vi "GetAllBooleanControls.vi"(8 "error in (no error)":errorcluster, 11 "VI in":refnum<vi>) -> (0 "error out":errorcluster, 3 "Boolean Controls":refnum<vi>[](array[refnum]))   [LabVIEW 2018, in "CarWashTestCases.lvclass"]
uses:
  CarWashTestCases.lvclass
  <vilib>/Utility/traverseref.llb/TRef TravTarget.ctl
  <vilib>/Utility/traverseref.llb/VI Scripting - Traverse.lvlib
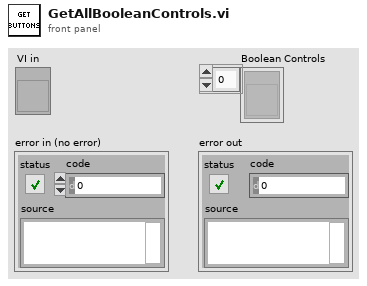
[diagram p1: front panel]
types:
  T1 = typedef "TRef TravTarget.ctl" = enum16{"FP", "BD", "Other"}
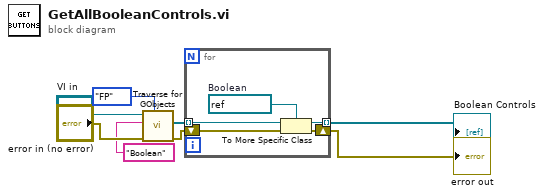
[diagram p0: block diagram]
diagram:
  n1 = call <vilib>:"Traverse for GObjects.vi"("Traverse Target"=TRef_TravTarget."FP", "error in (no error)"="error in (no error)", "Class Name"="Boolean", "VI Refnum"="VI in") -> ("error out"=w7:errorcluster, "References"=w4:refnum<vi>[])  [unwired: 4 in, 2 out]
  n2 = for {
    tunnel: w4 -> [w11] mode=indexing
    tunnel: [w12] -> w5 mode=indexing
    shift-right: [w9] -> w8
    shift-left: w7 -> [w10]
    w13 = refnum<vi> refnum  # Boolean
    n3 = To More Specific Class(target class=w13, reference=w11, error in=w10) -> (specific class reference=w12:refnum<vi>, error out=w9:errorcluster)
  }
  "error out" <- w8
  "Boolean Controls" <- w5
